vi "HW_Set_IO_Dir_on_ECU_2.vi"(2 "Error In":errorcluster, 4 "IO parameters cluster":T1, 5 "All Port Info":T3={"Type"=enum."Serial (VISA)", "Serial Port"="", "IP Address"="0.0.0.0"}) -> (0 "error out":errorcluster, 1 "Message":string)   [LabVIEW 2018, in "HW Interaction.lvlib"]
uses:
  HW Interaction.lvlib
  Public API/Typedefs/CTL_Port_connection_type.ctl
  SubVi's/Controls/CTL_IO_params_cluster.ctl
  Common_Resources.lvlib
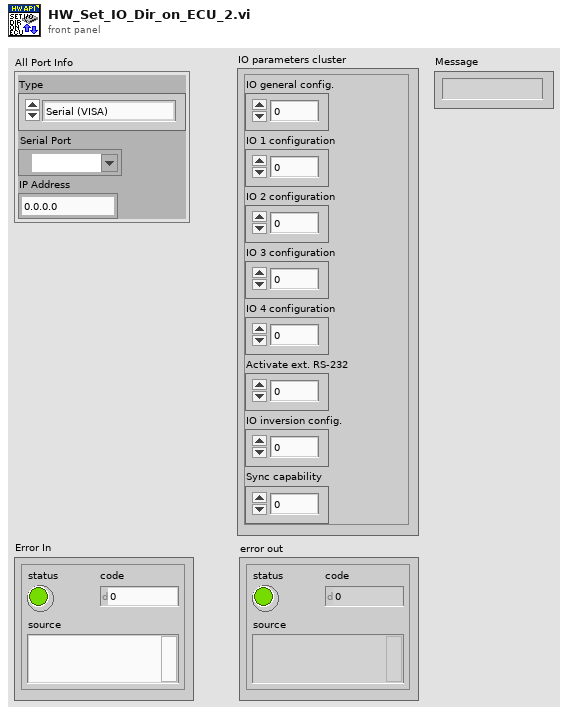
[diagram p1: front panel]
types:
  T1 = typedef "Common_Resources.lvlib/CTL_IO_params_cluster.ctl" = cluster{"IO general config.":u16, "IO 1 configuration":u16, "IO 2 configuration":u16, "IO 3 configuration":u16, "IO 4 configuration":u16, "Activate ext. RS-232":u16, "IO inversion config.":u16, "Sync capability":u8}
  T2 = typedef "HW Interaction.lvlib/CTL_Port_connection_type.ctl" = enum16{"Serial (VISA)", "TCP/IP"}
  T3 = cluster{"Type":T2, "Serial Port":refnum<visa-resource-name>, "IP Address":string}
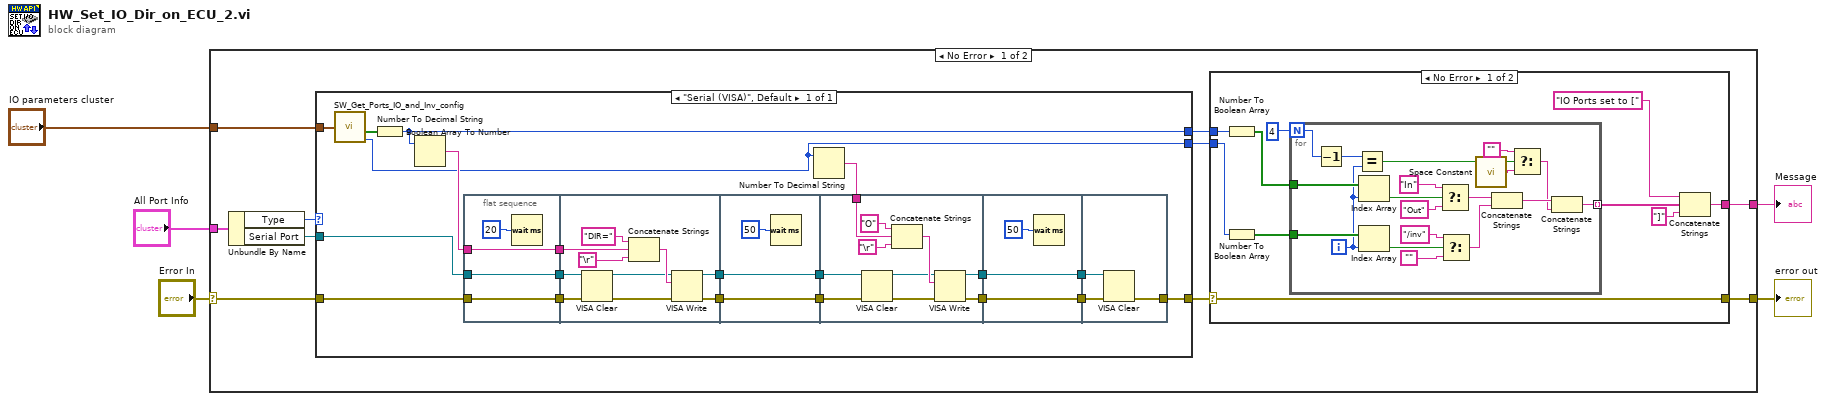
[diagram p0: block diagram]
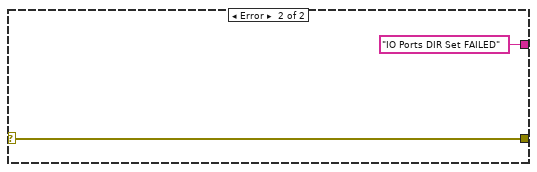
[diagram p2: hidden frame]
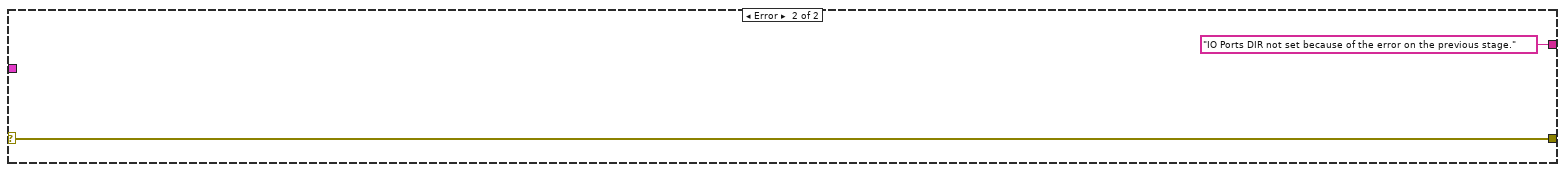
[diagram p3: hidden frame]
diagram:
  n1 = case shown="No Error" "Error In" {
    selector: "Error In" -> [w11 w101]
    tunnel: [w9 w101] -> w5
    tunnel: "IO parameters cluster" -> [w15 _]
    tunnel: "All Port Info" -> [w14 _]
    tunnel: [w8 "IO Ports DIR not set because of the error on the previous stage."] -> w1
    frame No Error {
      n2 = Unbundle By Name(w14) -> ("Type"=w13:T2, "Serial Port"=w12:refnum<visa-resource-name>)
      n3 = case shown="\"Serial (VISA)\", Default" w13 {
        tunnel: [w56] -> w10
        tunnel: w15 -> [w55]
        tunnel: w12 -> [w53]
        tunnel: w11 -> [w52]
        tunnel: [w51] -> w7
        tunnel: [w50] -> w6
        frame "Serial (VISA)", Default {
          n4 = call "SW_Get_Ports_IO_and_Inv_config.vi"("IO parameters cluster input"=w55) -> ("IO inversion config."=w50:u16, "Ports IO config (OUT is FALSE)"=w54:bool[])  [unwired: 3 out]
          n5 = Boolean Array To Number(Boolean array=w54) -> (number=w51:u32)
          n6 = Number To Decimal String(number=w51) -> (decimal integer string=w58:string)  [unwired: 1 in]
          n7 = flat-sequence {
            tunnel: w52 -> [w68]
            tunnel: w53 -> [w69]
            tunnel: w58 -> [w70]
            tunnel: [w70] -> w49
            tunnel: [w69] -> w48
            tunnel: [w68] -> w47
            tunnel: [w76] -> w66
            tunnel: [w75] -> w65
            tunnel: w49 -> [w73]
            tunnel: w48 -> [w72]
            tunnel: w47 -> [w71]
            tunnel: [w82] -> w64
            tunnel: w66 -> [w82]
            tunnel: [w81] -> w63
            tunnel: w65 -> [w81]
            tunnel: w57 -> [w88]
            tunnel: [w87] -> w62
            tunnel: [w86] -> w61
            tunnel: w64 -> [w85]
            tunnel: w63 -> [w84]
            tunnel: [w95] -> w60
            tunnel: w62 -> [w95]
            tunnel: [w94] -> w59
            tunnel: w61 -> [w94]
            tunnel: [w99] -> w56
            tunnel: w59 -> [w97]
            tunnel: w60 -> [w98]
            frame #0 {
              n8 = Wait (ms)(milliseconds to wait=u32 20) -> ()  [unwired: 1 out]
            }
            frame #1 {
              n9 = VISA Clear(VISA resource name=w72, error in (no error)=w71) -> (VISA resource name out=w78:refnum<visa-resource-name>, error out=w77:errorcluster)
              n10 = Concatenate Strings("DIR=" ("write buffer"), w73, "\r") -> (w80:string)
              n11 = VISA Write(VISA resource name=w78, write buffer=w80, error in (no error)=w77) -> (VISA resource name out=w76:refnum<visa-resource-name>, error out=w75:errorcluster)  [unwired: 1 out]
            }
            frame #2 {
              n12 = Wait (ms)(milliseconds to wait=u32 50) -> ()  [unwired: 1 out]
            }
            frame #3 {
              n13 = VISA Clear(VISA resource name=w85, error in (no error)=w84) -> (VISA resource name out=w89:refnum<visa-resource-name>, error out=w90:errorcluster)
              n14 = Concatenate Strings("O" ("write buffer"), w88, "\r") -> (w93:string)
              n15 = VISA Write(VISA resource name=w89, write buffer=w93, error in (no error)=w90) -> (VISA resource name out=w87:refnum<visa-resource-name>, error out=w86:errorcluster)  [unwired: 1 out]
            }
            frame #4 {
              n16 = Wait (ms)(milliseconds to wait=u32 50) -> ()  [unwired: 1 out]
            }
            frame #5 {
              n17 = VISA Clear(VISA resource name=w98, error in (no error)=w97) -> (error out=w99:errorcluster)  [unwired: 1 out]
            }
          }
          n18 = Number To Decimal String(number=w50) -> (decimal integer string=w57:string)  [unwired: 1 in]
        }
      }
      n19 = case shown="No Error" w10 {
        selector: w10 -> [w25 w46]
        tunnel: [w25 w46] -> w9
        tunnel: [w23 "IO Ports DIR Set FAILED"] -> w8
        tunnel: w7 -> [w22 _]
        tunnel: w6 -> [w21 _]
        frame No Error {
          n20 = Number To Boolean Array(number=w22) -> (Boolean array=w20:bool[])
          n21 = Number To Boolean Array(number=w21) -> (Boolean array=w19:bool[])
          n22 = for {
            N: 4 -> [w35]
            tunnel: w20 -> [w44]
            tunnel: w19 -> [w43]
            tunnel: [w31] -> w18 mode=indexing
            i -> [w33]
            n23 = Decrement(x=w35) -> (x-1=w34:i32)
            n24 = Equal?(x=w34, y=w33) -> (x = y?=w30:bool)
            n25 = Index Array(array=w44, index=w33) -> (element=w42:bool)
            n26 = Index Array(array=w43, index=w33) -> (element=w39:bool)
            n27 = Select(t="In", s=w42, f="Out") -> (s? t:f=w36:string)
            n28 = Select(t="/inv", s=w39, f="") -> (s? t:f=w26:string)
            n29 = call <vilib>:"Space Constant.vi"() -> ("String"=w27:string)
            n30 = Concatenate Strings(w36, w26) -> (w32:string)
            n31 = Select(t="", s=w30, f=w27) -> (s? t:f=w29:string)
            n32 = Concatenate Strings(w32, w29) -> (w31:string)
          }
          n33 = Concatenate Strings("IO Ports set to [", w18, "]" ("string")) -> (w23:string)
        }
        frame Error {
        }
      }
    }
    frame Error {
    }
  }
  "error out" <- w5
  "Message" <- w1
